vi "GUI Init - DOM.vi"(8 "error in (no error)":errorcluster, 9 "Ch.names":string[](array[string]), 10 "Cluster":T1, 11 "Array Ref.":refnum<vi>) -> (0 "error out":errorcluster, 2 "Data":dbl[](array[numeric]), 3 "Array Ref. out":refnum<vi>)   [LabVIEW 2017]
doc: "Initialize array's size and values for DOM Array by reference"
uses:
  Controls/Discrete_GUI_Cluster.ctl
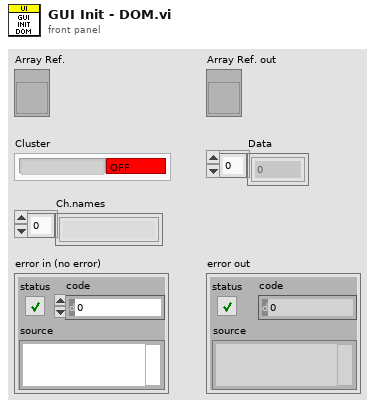
[diagram p1: front panel]
types:
  T1 = typedef "Discrete_GUI_Cluster.ctl" = cluster{"Ch.name":string, "Ch.state":bool}
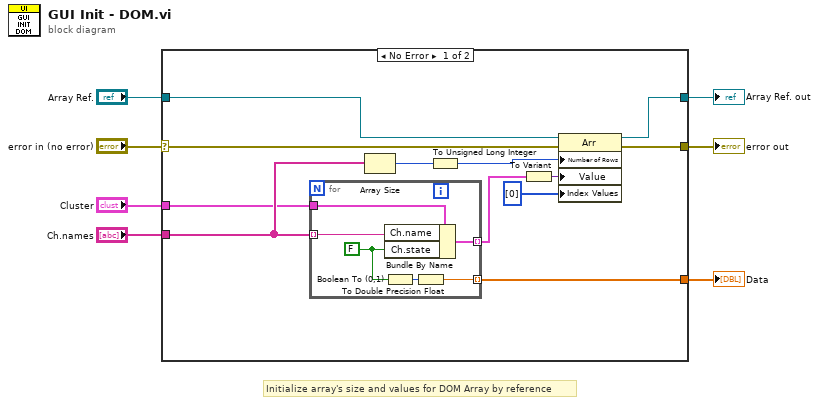
[diagram p0: block diagram]
diagram:
  # "Initialize array's size and values for DOM Array by reference"
  n1 = case shown="No Error" "error in (no error)" {
    selector: "error in (no error)" -> [w13 w27]
    tunnel: [w12 w27] -> w6
    tunnel: "Ch.names" -> [w16 _]
    tunnel: "Array Ref." -> [w15 w26]
    tunnel: "Cluster" -> [w14 _]
    tunnel: [w11 _] -> w3
    tunnel: [w8 w26] -> w1
    frame No Error {
      n2 = for {
        tunnel: [w25] -> w10 mode=indexing
        tunnel: w16 -> [w24] mode=indexing
        tunnel: w14 -> [w23]
        tunnel: [w20] -> w11 mode=indexing
        w21 = FALSE
        n3 = Bundle By Name(cluster=w23, "Ch.name"=w24, "Ch.state"=w21) -> (w25:T1)
        n4 = Boolean To (0,1)(Boolean=w21) -> (0, 1=w22:i16)
        n5 = To Double Precision Float(number=w22) -> (double precision float=w20:dbl)
      }
      n6 = Array Size(array=w16) -> (size(s)=w18:i32)
      n7 = To Unsigned Long Integer(number=w18) -> (unsigned 32bit integer=w17:u32)
      n8 = To Variant(anything=w10) -> (Variant=w9:variant)
      n9 = property class="Arr"(reference=w15, error in=w13, "Number of Rows"=w17, "Value"=w9, "Index Values"=u32[] [0]) -> (reference out=w8:refnum<vi>, error out=w12:errorcluster)
    }
    frame Error {
    }
  }
  "error out" <- w6
  "Data" <- w3
  "Array Ref. out" <- w1
